vi "Validate.vi"(8 "error in (no error)":errorcluster, 11 "Build in":refnum<class "AB_Targetfile.lvclass">) -> (0 "error out":errorcluster, 3 "Build out":refnum<class "AB_Targetfile.lvclass">)   [LabVIEW 2020, in "AB_Targetfile.lvclass"]
uses:
  <vilib>/AppBuilder/AB_Classes/TargetFile/AB_Targetfile.lvclass
  <vilib>/AppBuilder/AB_Classes/TargetFile/AB_Targetfile.lvclass/AB_Targetfile.ctl
  <resource>/Framework/Providers/Common/provcom_StringGlobals.vi
  <vilib>/AppBuilder/AB_Classes/Build/AB_Build.lvclass
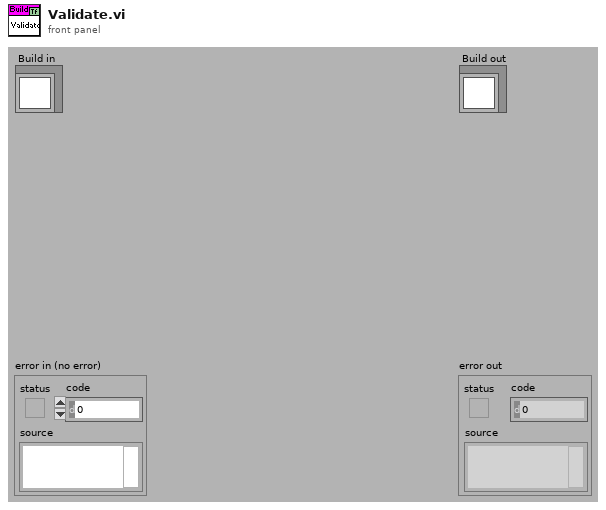
[diagram p1: front panel]
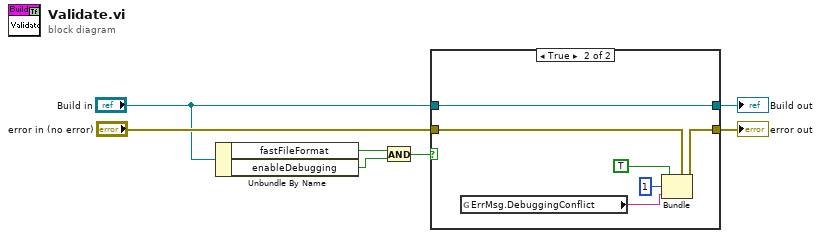
[diagram p0: block diagram]
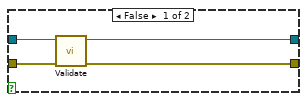
[diagram p2: hidden frame]
diagram:
  n1 = Unbundle By Name("Build in") -> ("fastFileFormat"=w3:bool, "enableDebugging"=w2:bool)
  n2 = And(x=w3, y=w2) -> (x .and. y?=w5:bool)
  n3 = case shown="True" w5 {
    tunnel: [w11 w12] -> w7
    tunnel: [w10 w17] -> w6
    tunnel: "error in (no error)" -> [w9 w13]
    tunnel: "Build in" -> [w8 w17]
    frame False {
      n4 = call-parent "Validate.vi"("error in (no error)"=w9, "Build in"=w8) -> ("error out"=w11:errorcluster, "Build out"=w10:refnum<class "AB_Targetfile.lvclass">)  [unwired: 8 in]
    }
    frame True {
      n5 = global read "provcom_StringGlobals.vi" "ErrMsg.DebuggingConflict"() -> (w14:string)
      n6 = Bundle(cluster=w13, "status"=TRUE, "code"=1, "source"=w14) -> (w12:errorcluster)
    }
  }
  "error out" <- w7
  "Build out" <- w6
